vi "Trial-duplicatepoints.vi"() -> ()   [LabVIEW 2019]
panel:
  out "Array":cluster{"x":i32, "y":i32}[](array[cluster])
  out "N Points":i32
  in  "y":i32
  in  "x":i32
  in  "OK Button":bool
  in  "Stop":bool
  out "XY Graph":cluster{"x":i32, "y":i32}[](graph)
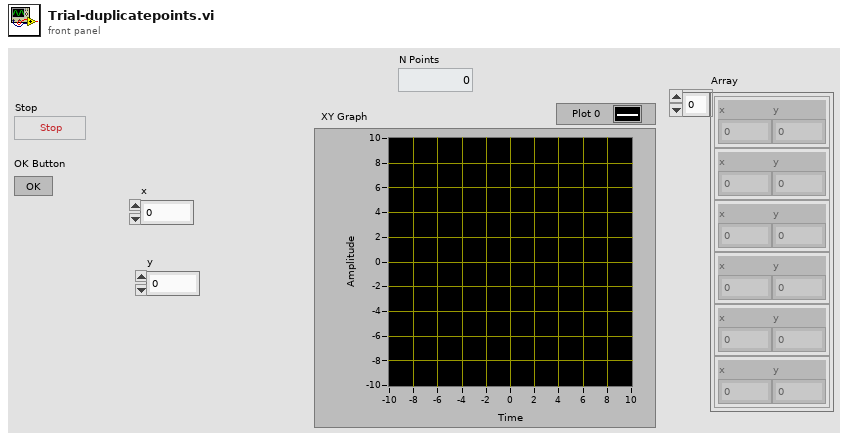
[diagram p1: front panel]
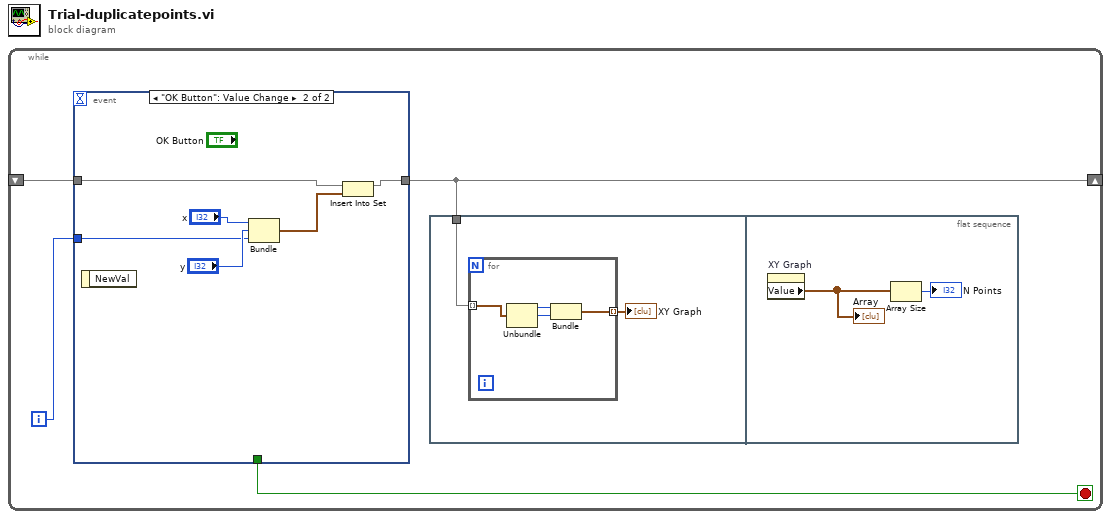
[diagram p0: block diagram]
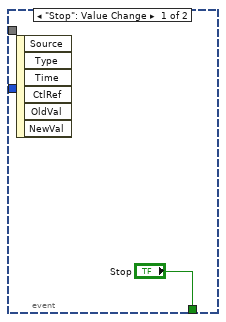
[diagram p2: hidden frame]
diagram:
  n1 = while {
    shift-right: [w1] -> _
    shift-left: _ -> [w2]
    i -> [w3]
    stop <- w4 stop-if-true
    n2 = event shown="[1] \"OK Button\": Value Change" {
      selector: _ -> [_ _]
      dyn-events: _ -> [_ _]
      timeout: _ -> [_ _]
      tunnel: ["Stop" _] -> w4
      tunnel: w3 -> [_ w17]
      tunnel: w2 -> [_ w16]
      tunnel: [_ w14] -> w1
      event "Stop": Value Change {
        n3 = event-data() -> ()  [unwired: 1 in, 6 out]
      }
      event "OK Button": Value Change {
        n4 = event-data() -> ()  [unwired: 1 in, 1 out]
        n5 = Bundle("x"="x", "y"="y", w17) -> (w15:cluster{"x":i32, "y":i32, i32})  [unwired: 1 in]
        n6 = Insert Into Set(10:w15, 11:w16) -> (3:w14:set{cluster{"x":i32, "y":i32, i32}})  [unwired: 1 out]
      }
    }
    n7 = flat-sequence {
      tunnel: w1 -> [w6]
      frame #0 {
        n8 = for {
          tunnel: w6 -> [w10] mode=indexing
          tunnel: [w7] -> w5 mode=indexing
          n9 = Unbundle(w10) -> ("x"=w9:i32, "y"=w8:i32)  [unwired: 1 out]
          n10 = Bundle("x"=w9, "y"=w8) -> (w7:cluster{"x":i32, "y":i32})  [unwired: 1 in]
        }
        "XY Graph" <- w5
      }
      frame #1 {
        n11 = property on="XY Graph" class="XYGraph (strict)"() -> ("Value"=w11:cluster{"x":i32, "y":i32}[])  [unwired: 2 in, 2 out]
        "Array" <- w11
        n12 = Array Size(array=w11) -> (size(s)=→"N Points":i32)
      }
    }
  }
